vi "Ack TCP Data.vi"(0 "connection ID":refnum<k5>, 3 "error in (no error)":errorcluster) -> (7 "connection ID out":refnum<k5>, 10 "error out":errorcluster)   [LabVIEW 2020]
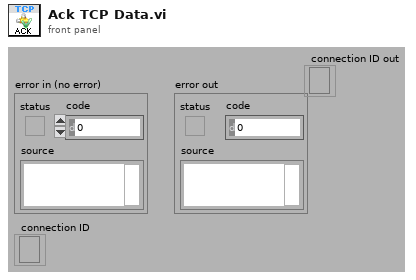
[diagram p1: front panel]
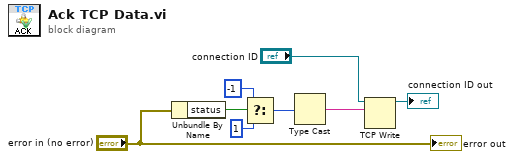
[diagram p0: block diagram]
diagram:
  n1 = Unbundle By Name("error in (no error)") -> ("status"=w7:bool)
  n2 = Select(t=-1, s=w7, f=1) -> (s? t:f=w4:i32)
  n3 = Type Cast(x=w4) -> (*(type *) &x=w8:string)  [unwired: 1 in]
  n4 = TCP Write(connection ID="connection ID", data in=w8) -> (connection ID out=→"connection ID out":refnum<k5>)  [unwired: 2 in, 2 out]
  "error out" <- "error in (no error)"
